vi "CoincidenceHistoGlobal.vi"(1 "set/change":bool, 2 "Array 2":T1(array[cluster]) {"offset (ns)" format="%.2f"; "origin (ns)" format="%.2f"}) -> (0 "Array":T1(array[cluster]) {"offset (ns)" format="%.2f"; "origin (ns)" format="%.2f"})   [LabVIEW 2009]
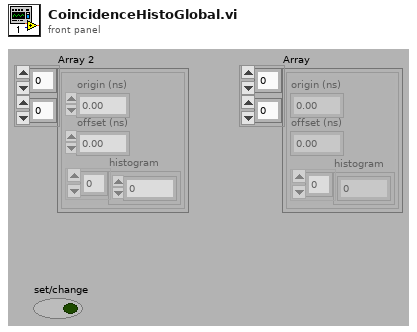
[diagram p1: front panel]
types:
  T1 = cluster{"origin (ns)":dbl, "offset (ns)":dbl, "histogram":u32[]}[][]
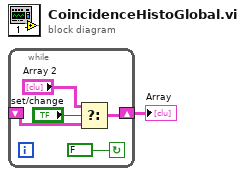
[diagram p0: block diagram]
diagram:
  n1 = while {
    shift-right: [w4] -> w1
    shift-left: _ -> [w5]
    stop <- FALSE continue-if-true
    n2 = Select(t="Array 2", s="set/change", f=w5) -> (s? t:f=w4:T1)
  }
  "Array" <- w1
